vi "ЛР4 - 1 варик.vi"() -> ()   [LabVIEW 2012]
uses:
  <vilib>/Analysis/NI_AALPro.lvlib
  <vilib>/Analysis/NI_AALBase.lvlib
panel:
  in  "Out":bool
  out "Waveform Graph":dbl[](graph)
  in  "?":bool
  in  "?":dbl(slide) scale=100.0..1000.0
  in  "Noise amplitude":dbl(knob) scale=0.0..3.0
  in  "Signal type":T1(ring)
  in  "Samples":i32
  in  "Noise":u16(ring) items=["Uniform White", "Periodic Random", "Poisson Noise "]
  in  "Square wave duty cycle (%)":dbl
  in  "Sine frequency":dbl(slide) scale=10.0..100.0
  in  "Frequency":dbl(knob) scale=0.0..10.0
  in  "Amplitude":dbl(slide) scale=0.0..10.0
  # "Radio imp"
  # "Video imp"
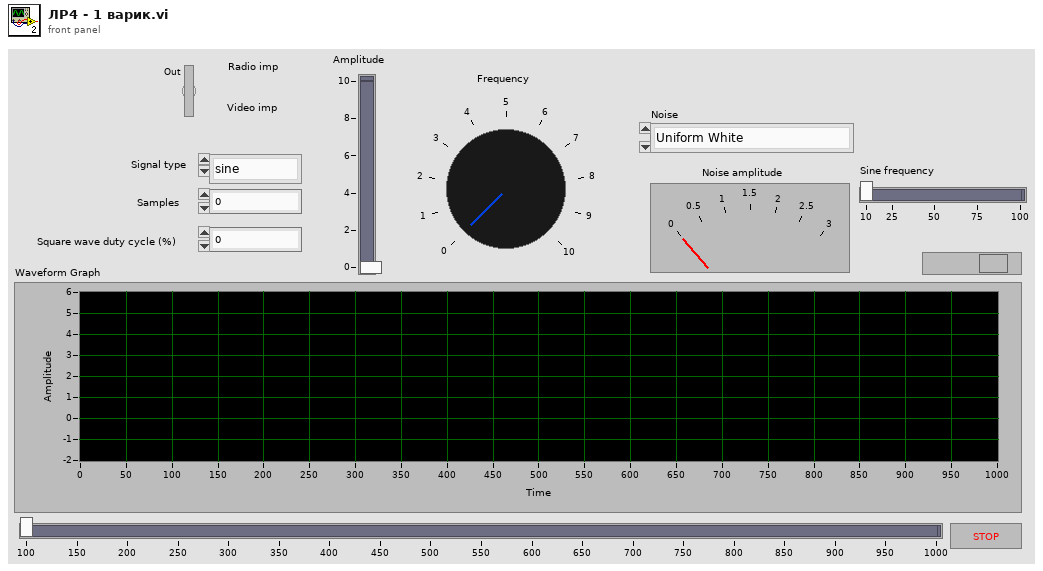
[diagram p1: front panel]
types:
  T1 = enum16{"sine", "cosine", "triangle", "square", "sawtooth", "increasing ramp", "decreasing ramp"}
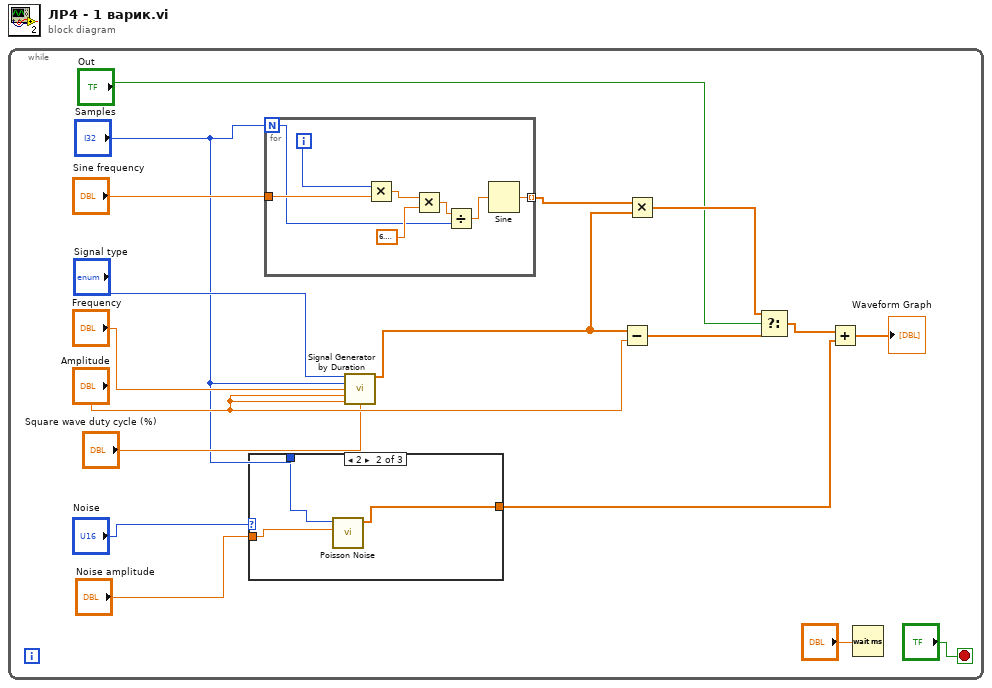
[diagram p0: block diagram]
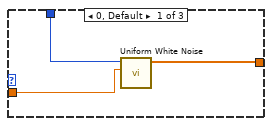
[diagram p2: hidden frame]
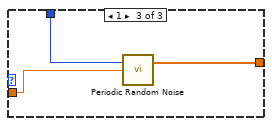
[diagram p3: hidden frame]
diagram:
  n1 = while {
    stop <- "?" stop-if-true
    n2 = case shown="2" "Noise" {
      tunnel: "Samples" -> [w21 w23 w27]
      tunnel: "Noise amplitude" -> [w20 w24 w25]
      tunnel: [w19 w22 w26] -> w7
      frame 0, Default {
        n3 = call <vilib>:"Uniform White Noise.vi"("amplitude"=w20, "samples"=w21) -> ("uniform white noise"=w19:dbl[])  [unwired: 8 in, 1 out]
      }
      frame 2 {
        n4 = call <vilib>:"Poisson Noise.vi"("mean"=w24, "samples"=w23) -> ("poisson noise"=w22:dbl[])  [unwired: 8 in, 1 out]
      }
      frame 1 {
        n5 = call <vilib>:"Periodic Random Noise.vi"("spectral amplitude"=w25, "samples"=w27) -> ("periodic random noise"=w26:dbl[])  [unwired: 1 in, 1 out]
      }
    }
    n6 = for {
      N: "Samples" -> [w28]
      tunnel: [w33] -> w6 mode=indexing
      tunnel: "Sine frequency" -> [w35]
      i -> [w34]
      n7 = Multiply(x=w34, y=w35) -> (x*y=w32:dbl)
      n8 = Multiply(x=w32, y=6.283185307179586) -> (x*y=w30:dbl)
      n9 = Divide(x=w30, y=w28) -> (x/y=w29:dbl)
      n10 = Sine(x=w29) -> (sin(x)=w33:dbl)
    }
    n11 = call <vilib>:"Signal Generator by Duration.vi"("signal type"="Signal type", "# of samples"="Samples", "frequency"="Frequency", "amplitude"="Amplitude", "dc offset"="Amplitude", "square wave duty cycle (%)"="Square wave duty cycle (%)") -> ("signal"=w5:dbl[])  [unwired: 6 in, 3 out]
    n12 = Subtract(x=w5, y="Amplitude") -> (x-y=w16:dbl[])
    n13 = Multiply(x=w6, y=w5) -> (x*y=w17:dbl[])
    n14 = Select(t=w17, s="Out", f=w16) -> (s? t:f=w15:dbl[])
    n15 = Add(x=w15, y=w7) -> (x+y=→"Waveform Graph":dbl[])
    n16 = Wait (ms)(milliseconds to wait="?") -> ()  [unwired: 1 out]
  }
